vi "Lorentzian test.vi"(3 "output control":T1, 4 "data":variant, 5 "X":dbl[](array[numeric]), 6 "a":dbl[](array[numeric])) -> (0 "error out":errorcluster, 1 "f'(X,a)":dbl[][](array[numeric]), 2 "f(X,a)":dbl[](array[numeric]))   [LabVIEW 2016]
doc: "Sum of three Gaussians, plus DC offset."
uses:
  <vilib>/gmath/NumericalOptimization/LM_output select.ctl
  <vilib>/gmath/NI_Gmath.lvlib
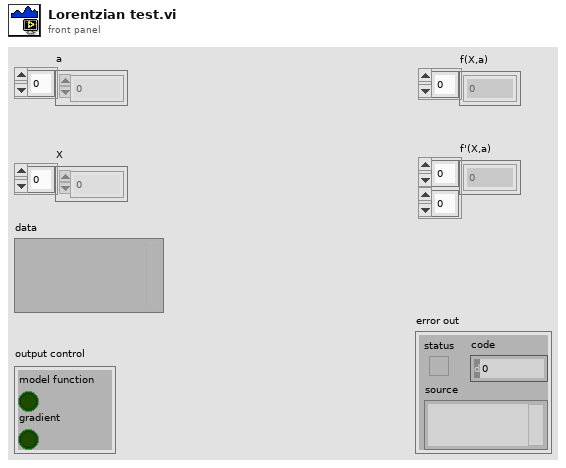
[diagram p1: front panel]
types:
  T1 = typedef "NI_Gmath.lvlib/LM_output select.ctl" = cluster{"model function":bool, "gradient":bool}
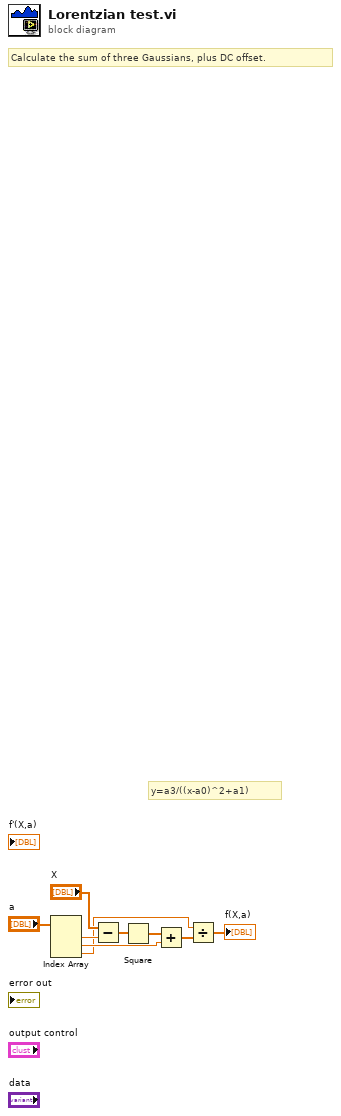
[diagram p0: block diagram]
diagram:
  # "y=a3/((x-a0)^2+a1)"
  # "Calculate the sum of three Gaussians, plus DC offset."
  n1 = Index Array(array="a") -> (element #1=w7:dbl, element #2=w5:dbl, element #3=w3:dbl)  [unwired: 3 in]
  n2 = Subtract(x="X", y=w7) -> (x-y=w6:dbl[])
  n3 = Square(x=w6) -> (x^2=w1:dbl[])
  n4 = Add(x=w1, y=w5) -> (x+y=w4:dbl[])
  n5 = Divide(x=w3, y=w4) -> (x/y=→"f(X,a)":dbl[])
